vi "Close.vi"(8 "error in (no error)":errorcluster, 11 "reference in":refnum<class "TestView_Tree_Single.lvclass">) -> (0 "error out":errorcluster, 3 "reference in":refnum<class "TestView_Tree_Single.lvclass">)   [LabVIEW 2022 SP3, in "TestView_Tree_Single.lvlib" / "TestView_Tree_Single.lvclass"]
uses:
  TestView_Tree_Single.lvclass
  Components/TestView_Base.lvlibp/TestView_Base.lvclass
  Components/ViPER.lvlibp/ViPER.lvclass
  C:/Projects/Medulla/ViPER/Examples/Flux_Capacitor_Tester/Components/ViPER.lvlibp/ViPER.lvclass
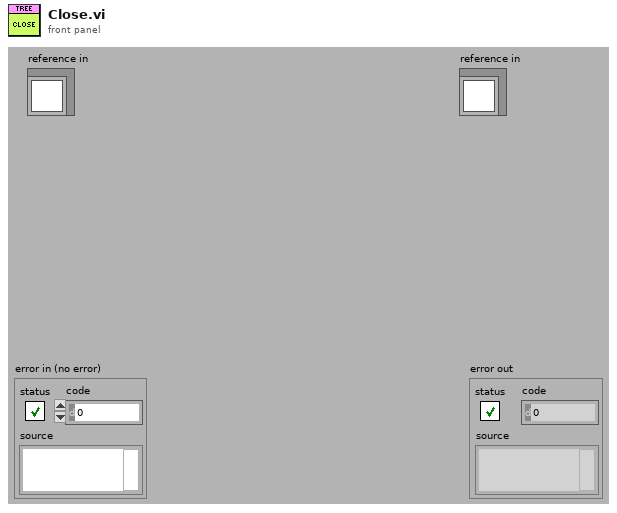
[diagram p1: front panel]
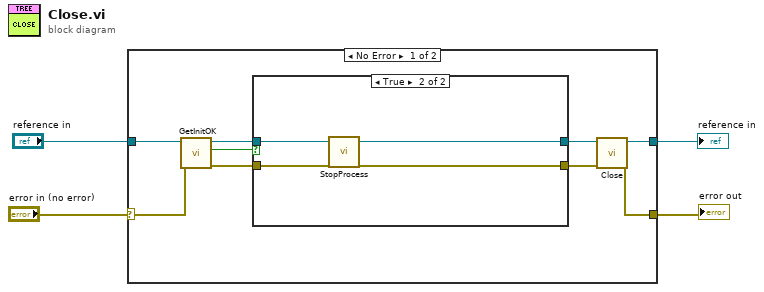
[diagram p0: block diagram]
diagram:
  n1 = case shown="No Error" "error in (no error)" {
    selector: "error in (no error)" -> [w8 w21]
    tunnel: [w13 w21] -> w3
    tunnel: [w12 w20] -> w1
    tunnel: "reference in" -> [w9 w20]
    frame No Error {
      n2 = call "GetInitOK.vi"("error in (no error)"=w8, "reference in"=w9) -> ("error out"=w5:errorcluster, "init_ok"=w6:bool, "reference out"=w7:refnum<class "TestView_Tree_Single.lvclass">)  [unwired: 7 in]
      n3 = case shown="True" w6 {
        tunnel: [w15 w19] -> w11
        tunnel: [w14 w16] -> w10
        tunnel: w7 -> [w15 w18]
        tunnel: w5 -> [w14 w17]
        frame False {
        }
        frame True {
          n4 = call "StopProcess.vi"("reference in"=w18, "error in (no error)"=w17) -> ("reference out"=w19:refnum<class "TestView_Tree_Single.lvclass">, "error out"=w16:errorcluster)  [unwired: 16 in]
        }
      }
      n5 = call-parent "Close.vi"("error in (no error)"=w10, "reference in"=w11) -> ("error out"=w13:errorcluster, "reference in"=w12:refnum<class "TestView_Tree_Single.lvclass">)  [unwired: 8 in]
    }
    frame Error {
    }
  }
  "error out" <- w3
  "reference in" <- w1
